vi "ConfigAndFilters.vi"(9 "Limit":enum16{""}(ring), 10 "Sensor":enum16{""}(ring), 11 "Device":enum16{""}(ring)) -> ()   [LabVIEW 2026]
panel:
  # "Konfiguracja i filtry"
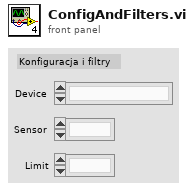
[diagram p1: front panel]
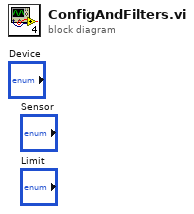
[diagram p0: block diagram]
diagram:
